vi "_Add Metrics.vi"(8 "error in (no error)":errorcluster, 10 "Metrics":refnum<data-value>[](array[refnum]), 11 "Default Collector in":refnum<class "Default Collector.lvclass">) -> (0 "error out":errorcluster, 3 "Default Collector out":refnum<class "Default Collector.lvclass">)   [LabVIEW 2020, in "Collector.lvlib" / "Default Collector.lvclass"]
uses:
  Default Collector.lvclass
  metrics/metric/Metric.lvclass
  Default Collector.lvclass/Default Collector.ctl
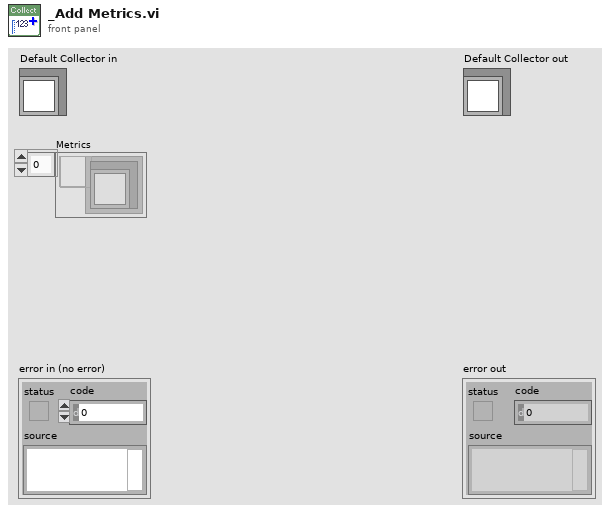
[diagram p1: front panel]
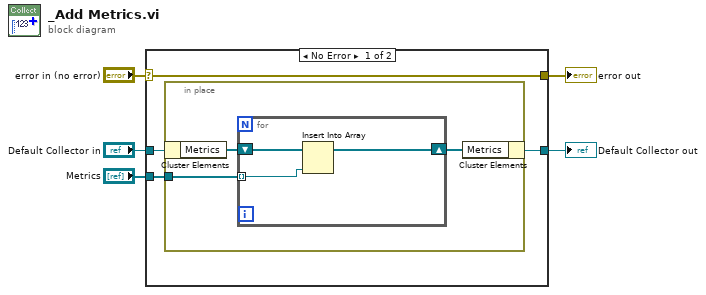
[diagram p0: block diagram]
diagram:
  n1 = case shown="No Error" "error in (no error)" {
    selector: "error in (no error)" -> [w9 w17]
    tunnel: [w9 w17] -> w4
    tunnel: [w6 w16] -> w2
    tunnel: "Default Collector in" -> [w8 w16]
    tunnel: "Metrics" -> [w7 _]
    frame No Error {
      n2 = in-place {
        in-place-border: w7 -> [w11]
        n3 = in-place-cluster #1(w8) -> ("Metrics"=w12:refnum<data-value>[])
        n4 = for {
          tunnel: w11 -> [w14] mode=indexing
          shift-right: [w13] -> w10
          shift-left: w12 -> [w15]
          n5 = Insert Into Array(array=w15, new element=w14) -> (w13:refnum<data-value>[])  [unwired: 1 in]
        }
        n6 = in-place-cluster #1("Metrics"=w10) -> (w6:refnum<class "Default Collector.lvclass">)
      }
    }
    frame Error {
    }
  }
  "error out" <- w4
  "Default Collector out" <- w2
